vi "Solenoid - Fill.vi"(7 "Semiphore":T1, 8 "Error In":errorcluster, 10 "VALVE OPEN CLOSE":enum8{"OPEN", "CLOSE"}(ring), 11 "VISA session":refnum<visa-resource-name>="MW100") -> (0 "Error Out":errorcluster, 3 "dup VISA session":refnum<visa-resource-name>)   [LabVIEW 2012]
uses:
  ChannelSettings.ctl
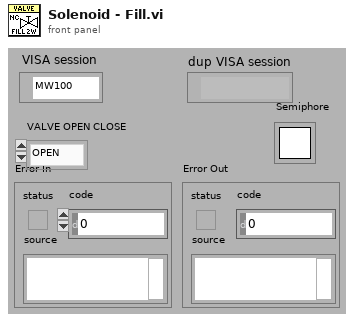
[diagram p1: front panel]
types:
  T1 = typedef "Semaphore RefNum" = refnum<k1>
  T2 = typedef "ChannelSettings.ctl" = u32
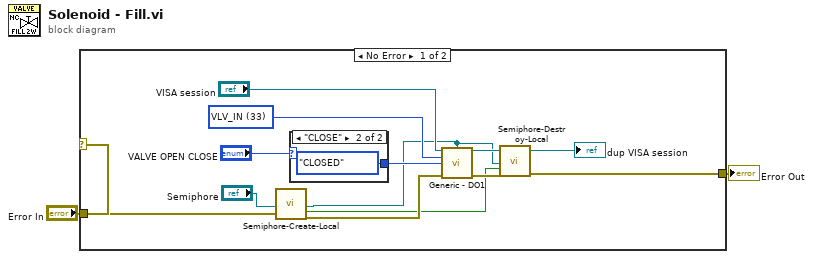
[diagram p0: block diagram]
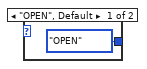
[diagram p2: hidden frame]
diagram:
  n1 = case shown="No Error" "Error In" {
    selector: "Error In" -> [_ w17]
    tunnel: "Error In" -> [w10 _]
    tunnel: [w5 w17] -> w2
    frame No Error {
      w8 = T2 33 items=["4-20_OUT", "Pres_HI1", "Pres_HI2", "Pres_LOW", "Pres_PIN", "HEATER_TOP", "HEATER_BOT", "T_Shell", "FLOWMETER", "WATT_SENSE", "WH_TICK", "Tc_1", "Tc_2", "Tc_3", "Tc_4", "Tc_5", "Tc_6", "Tc_down", "T_Shell_2", "T_Shell_3", "T_Shell_4", "RTD_IN", "RTD_OUT", "RTD_AMB", "INTF_TEMPFLO", "INTF_READY", "INTF_START", "INTF_STOP", "DRM_LOW", "DRM_HIGH", "PWR_MAIN", "VLV_DUMP", "VLV_OUT", "VLV_IN", "WATT_HOURS", "FLOW(SAMPLE)", "GALLONS", "FLOW(GPM)"] ("Channel_Enum")
      n2 = call "Semiphore-Create-Local.vi"("Semiphore"="Semiphore", "error in (no error)"=w10) -> ("semaphore"=w4:T1, "Local?"=w3:bool, "error out"=w9:errorcluster)  [unwired: 15 in]
      n3 = case shown="\"CLOSE\"" "VALVE OPEN CLOSE" {
        tunnel: [enum8{"CLOSED", "OPEN"}."OPEN" ("Relay Status (0:CLOSED)") enum8{"CLOSED", "OPEN"}."CLOSED" ("Relay Status (0:CLOSED)")] -> w11
        frame "OPEN", Default {
        }
        frame "CLOSE" {
        }
      }
      n4 = call "Generic - DO1.vi"("VISA session"="VISA session", "Semiphore"=w4, "Channel_Enum"=w8, "Relay Status (0:CLOSED)"=w11, "Error In"=w9) -> ("dup VISA session"=→"dup VISA session":refnum<visa-resource-name>, "error out"=w6:errorcluster)  [unwired: 9 in]
      n5 = call "Semiphore-Destroy-Local.vi"("Semiphore"=w4, "Local?"=w3, "error in (no error)"=w6) -> ("error out"=w5:errorcluster)  [unwired: 16 in]
    }
    frame Error {
    }
  }
  "Error Out" <- w2
